vi "Changer.vi"(0 "toChanger":T1(array[cluster]), 1 "out":i8[](array[numeric]), 2 "in":i8[](array[numeric])) -> ()   [LabVIEW 2017]
panel:
  out "error out":errorcluster
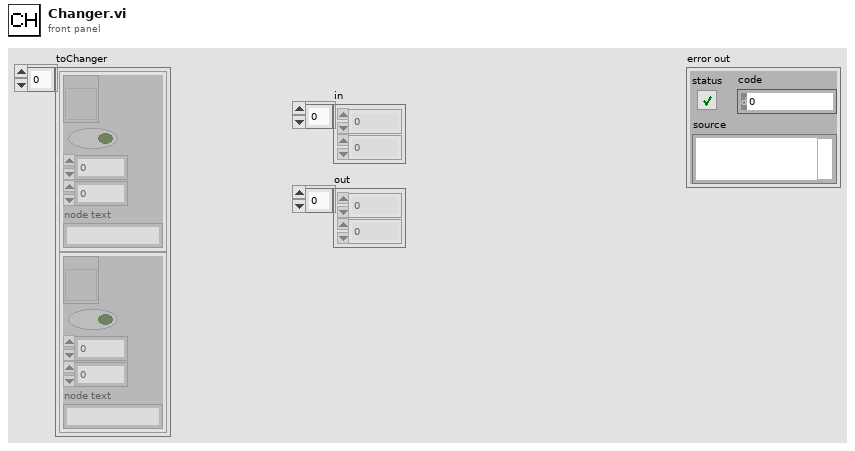
[diagram p1: front panel]
types:
  T1 = cluster{refnum<vi>, bool, i32, i32, "node text":string}[]
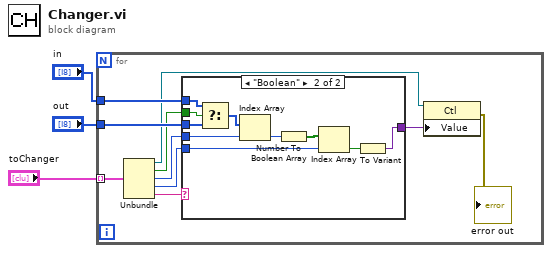
[diagram p0: block diagram]
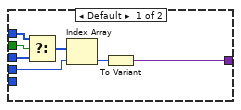
[diagram p2: hidden frame]
diagram:
  n1 = for {
    tunnel: "out" -> [w13]
    tunnel: "toChanger" -> [w12] mode=indexing
    tunnel: "in" -> [w10]
    n2 = Unbundle(w12) -> (w6:refnum<vi>, w9:bool, w8:i32, w11:i32, "node text"=w7:string)
    n3 = case shown="\"Boolean\"" w7 {
      tunnel: w13 -> [w20 w29]
      tunnel: [w18 w25] -> w5
      tunnel: w11 -> [_ w24]
      tunnel: w10 -> [w17 w23]
      tunnel: w9 -> [w16 w22]
      tunnel: w8 -> [w15 w21]
      frame Default {
        n4 = Select(t=w17, s=w16, f=w20) -> (s? t:f=w19:i8[])
        n5 = Index Array(array=w19, index=w15) -> (element=w14:i8)
        n6 = To Variant(anything=w14) -> (Variant=w18:variant)
      }
      frame "Boolean" {
        n7 = Select(t=w23, s=w22, f=w29) -> (s? t:f=w28:i8[])
        n8 = Index Array(array=w28, index=w21) -> (element=w27:i8)
        n9 = Number To Boolean Array(number=w27) -> (Boolean array=w30:bool[])
        n10 = Index Array(array=w30, index=w24) -> (element=w26:bool)
        n11 = To Variant(anything=w26) -> (Variant=w25:variant)
      }
    }
    n12 = property on="Property Node" class="Ctl"(reference=w6, "Value"=w5) -> (error out=→"error out":errorcluster)  [unwired: 1 in, 1 out]
  }
